vi "Add Default Free.vi"(8 "error in (no error)":errorcluster, 10 "ToModBus":bool, 11 "Dyn In":refnum<class "Dynamic.lvclass">) -> (0 "error out":errorcluster, 3 "Dyn Out":refnum<class "Dynamic.lvclass">)   [LabVIEW 2018, in "Measurement Channels.lvlib" / "Dynamic.lvclass"]
uses:
  Dynamic.lvclass
  Dynamic.lvclass/Dynamic.ctl
  Class Voltage/Voltage.lvclass
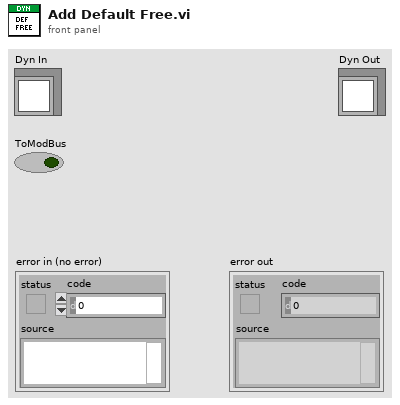
[diagram p1: front panel]
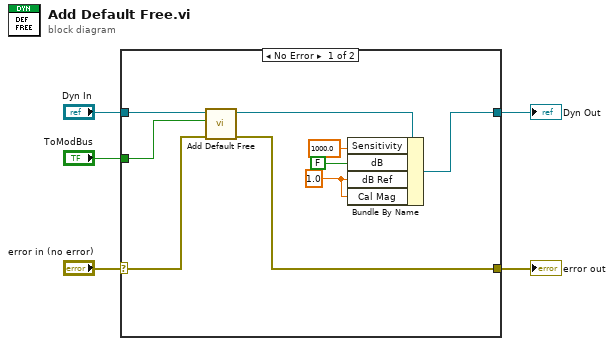
[diagram p0: block diagram]
diagram:
  n1 = case shown="No Error" "error in (no error)" {
    selector: "error in (no error)" -> [w6 w15]
    tunnel: "Dyn In" -> [w14 w16]
    tunnel: [w12 w16] -> w4
    tunnel: [w11 w15] -> w3
    tunnel: "ToModBus" -> [w7 _]
    frame No Error {
      w8 = 1.0 ("dB Ref")
      n2 = call-parent "Add Default Free.vi"("error in (no error)"=w6, "ToModBus"=w7, "Volt In"=w14) -> ("error out"=w11:errorcluster, "Volt Out"=w13:refnum<class "Dynamic.lvclass">)  [unwired: 7 in]
      n3 = Bundle By Name(cluster=w13, "Sensitivity"=1000.0, "dB"=FALSE, "dB Ref"=w8, "Cal Mag"=w8) -> (w12:refnum<class "Dynamic.lvclass">)
    }
    frame Error {
    }
  }
  "Dyn Out" <- w4
  "error out" <- w3
